vi "setUp.vi"(8 "error in (no error)":errorcluster, 11 "reference in":refnum<class "%DEVICE% Messaging Tests.lvclass">) -> (0 "error out":errorcluster, 3 "reference out":refnum<class "%DEVICE% Messaging Tests.lvclass">)   [LabVIEW 2017, in "%DEVICE% Messaging Tests.lvclass"]
doc: "setUp runs prior to the test method during test execution. Use this method to initialize any object data required by your tests."
uses:
  %DEVICE% Messaging Tests.lvclass
  C:/Program Files (x86)/National Instruments/LabVIEW 2017/vi.lib/addons/_JKI Toolkits/VI Tester/TestCase.llb/TestCase.lvclass
  Includes/CDMessaging.lvlibp/Producer/Abstract Producer/Abstract Producer.lvclass
  Includes/CDMessaging.lvlibp/Parameters/Abstract Init Parameters/Abstract Init Parameters.lvclass
  NI-SWITCH Init Parameters/NI-SWITCH Init Parameters.lvclass
  C:/Users/Admin/Documents/niveristand-routing-and-faulting-message-library/Includes/CDMessaging.lvlibp/Parameters/Abstract Init Parameters/Abstract Init Parameters.lvclass
  C:/Users/Admin/Documents/niveristand-routing-and-faulting-message-library/Includes/CDMessaging.lvlibp/Switch/Abstract Switch Init Parameters/Abstract Switch Init Parameters.lvclass
  Includes/CDMessaging.lvlibp/Message Queue/Message Queue/Message Queue.lvclass
  C:/Users/Admin/Documents/niveristand-routing-and-faulting-message-library/Includes/CDMessaging.lvlibp/Message Queue/Abstract Message Queue/Abstract Message Queue.lvclass
  Support/Mock %DEVICE% Consumer.lvclass
  C:/Users/Admin/Documents/niveristand-routing-and-faulting-message-library/Includes/CDMessaging.lvlibp/Switch/Abstract Switch Consumer/Abstract Switch Consumer.lvclass
  %DEVICE% Messaging Tests.lvclass/%DEVICE% Messaging Tests.ctl
  <vilib>/addons/_JKI Toolkits/VI Tester/TestCase.llb/TestCase.lvclass
  Includes/CDMessaging.lvlibp/Consumer/Abstract Consumer/Abstract Consumer.lvclass
  C:/Users/Admin/Documents/niveristand-routing-and-faulting-message-library/Includes/CDMessaging.lvlibp/Consumer/Abstract Consumer/Abstract Consumer.lvclass
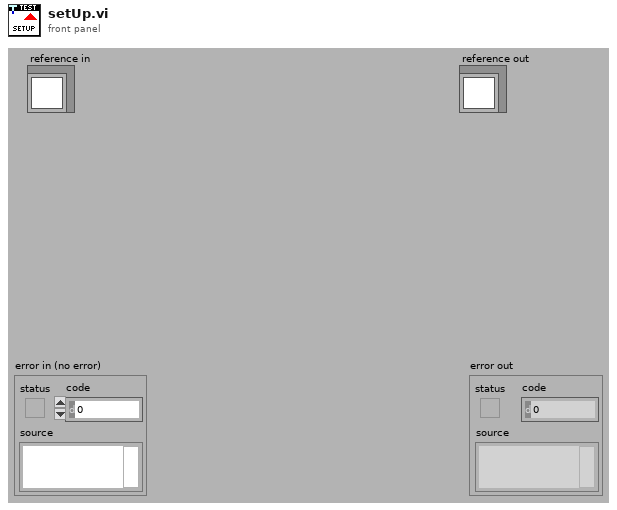
[diagram p1: front panel]
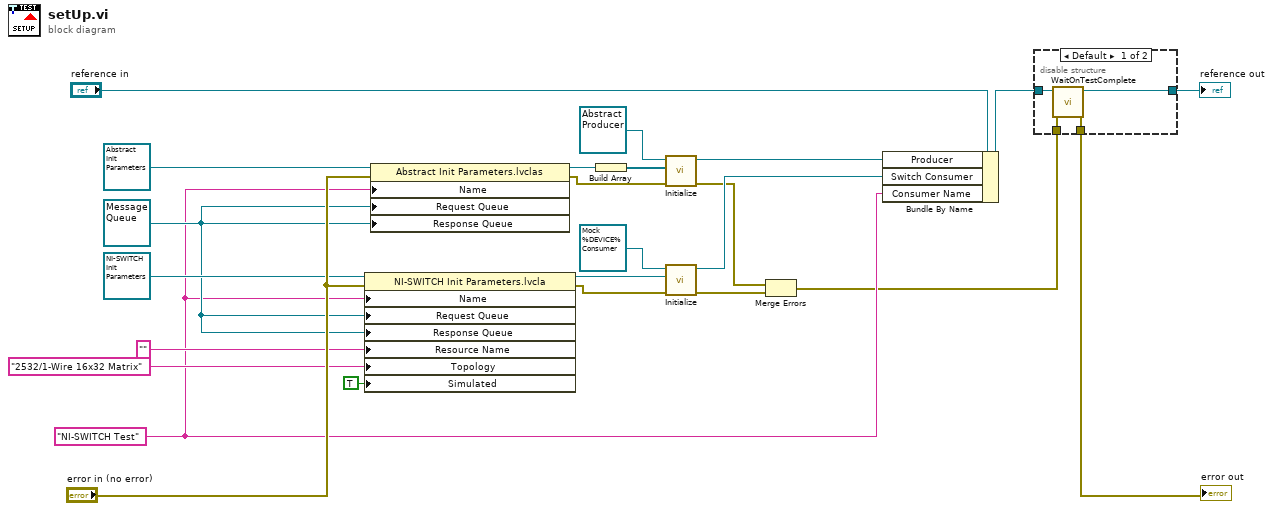
[diagram p0: block diagram]
diagram:
  w7 = "NI-SWITCH Test"
  w17 = refnum<class "Message Queue.lvclass"> refnum ("CDMessaging.lvlibp:Message Queue.lvclass")
  n1 = property class="NI-SWITCH Init Parameters.lvcla"(reference=refnum<class "NI-SWITCH Init Parameters.lvclass"> refnum ("SLSC Switch Messaging.lvlib:SLSC Switch Init Parameters.lvclass"), error in="error in (no error)", "Name"=w7, "Request Queue"=w17, "Response Queue"=w17, "Resource Name"="", "Topology"="2532/1-Wire 16x32 Matrix", "Simulated"=TRUE) -> (reference out=w10:refnum<class "NI-SWITCH Init Parameters.lvclass">, error out=w5:errorcluster)
  n2 = property class="Abstract Init Parameters.lvclas"(reference=refnum<class "Abstract Init Parameters.lvclass"> refnum ("CDMessaging.lvlibp:Abstract Init Parameters.lvclass"), error in="error in (no error)", "Name"=w7, "Request Queue"=w17, "Response Queue"=w17) -> (reference out=w13:refnum<class "Abstract Init Parameters.lvclass">, error out=w4:errorcluster)
  n3 = Build Array(w13) -> (w12:refnum<class "Abstract Init Parameters.lvclass">[])
  n4 = call "Initialize.vi"("error in (no error)"=w4, "Parameters in"=w12, "Abstract Producer in"=refnum<class "Abstract Producer.lvclass"> refnum ("CDMessaging.lvlibp:Abstract Producer.lvclass")) -> ("error out"=w3:errorcluster, "Abstract Producer out"=w9:refnum<class "Abstract Producer.lvclass">)  [unwired: 7 in]
  n5 = call "Initialize.vi"("error in (no error)"=w5, "Parameters in"=w10, "Abstract Consumer in"=refnum<class "Mock %DEVICE% Consumer.lvclass"> refnum ("Mock NI-SWITCH Consumer.lvclass")) -> ("error out"=w2:errorcluster, "Abstract Consumer out"=w8:refnum<class "Mock %DEVICE% Consumer.lvclass">)  [unwired: 7 in]
  n6 = Merge Errors(w3, w2) -> (w1:errorcluster)
  n7 = Bundle By Name(cluster="reference in", "Producer"=w9, "Switch Consumer"=w8, "Consumer Name"=w7) -> (w20:refnum<class "%DEVICE% Messaging Tests.lvclass">)
  n8 = disable-structure shown="Default" {
    disable-tunnel: w1 -> [w28 w29]
    disable-tunnel: [w27 w29] -> w23
    disable-tunnel: [w26 w30] -> w21
    disable-tunnel: w20 -> [w25 w30]
    frame condition #0 (active) {
      n9 = call <vilib>:"WaitOnTestComplete.vi"("error in (no error)"=w28, "TestCase in"=w25) -> ("error out"=w27:errorcluster, "TestCase out"=w26:refnum<class "%DEVICE% Messaging Tests.lvclass">)  [unwired: 8 in]
    }
    frame condition #1 {
    }
  }
  "error out" <- w23
  "reference out" <- w21
